vi "MCL Get Commanded Position.vi"(7 "handle":i32, 8 "error in (no error)":errorcluster, 9 "zCom":dbl, 10 "yCom":dbl, 11 "xCom":dbl) -> (0 "error out":errorcluster, 1 "zCom out":dbl, 2 "yCom out":dbl, 3 "xCom out":dbl, 5 "function return":i32)   [LabVIEW 2014, in "Madlib.lvlib"]
doc: "MADLIB_API int MCL_GetCommandedPosition(double *xCom, double *yCom, double *zCom, int handle);"
uses:
  <userlib>/Lambda2/lib/Madlib/Madlib.lvlib
  <userlib>/Lambda2/lib/Madlib/Madlib.dll
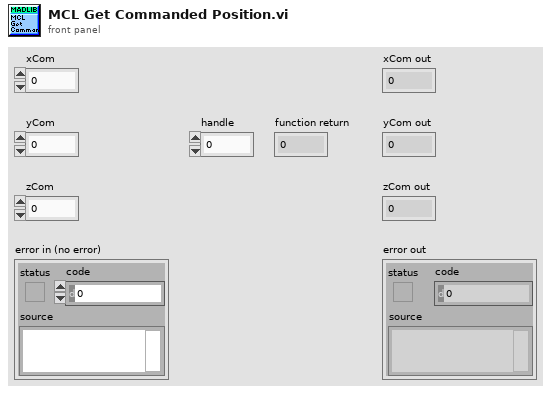
[diagram p1: front panel]
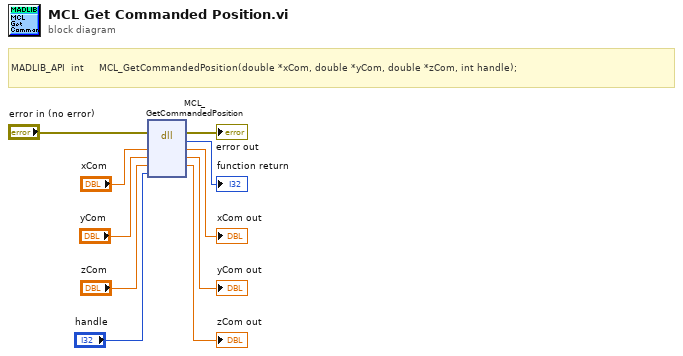
[diagram p0: block diagram]
diagram:
  # "MADLIB_API  int     MCL_GetCommandedPosition(double *xCom, double *yCom, double *zCom, int handle);"
  n1 = dll-call lib="C:/Program Files (x86)/National Instruments/LabVIEW 2014/user.lib/Lambda2/lib/Madlib/Madlib.*" fn="MCL_GetCommandedPosition"(error in="error in (no error)", "xCom"="xCom", "yCom"="yCom", "zCom"="zCom", "handle"="handle") -> (error out=→"error out":errorcluster, →"function return":i32, "xCom"=→"xCom out":dbl, "yCom"=→"yCom out":dbl, "zCom"=→"zCom out":dbl)  [unwired: 3 in, 1 out]
